vi "vPage_9237x1_CHx4.vi"() -> ()   [LabVIEW 2022 SP3]
uses:
  <vilib>/Utility/sysdir.llb/System Directory Type.ctl
panel:
  in  "Show_FFT":bool
  out "C2":i32
  out "DAQ Stoped":bool
  out "C1":i32
  in  "SW \n(C1)":bool[](array[boolean])=[TRUE, TRUE, TRUE, TRUE, TRUE, TRUE, TRUE, TRUE]
  in  "Sample \nto Read":i32=2000
  in  "Sample\nRate":dbl=2000.0
  in  "¸ê®Æ§¨\nµù°O>":string
  in  "Enable Saving":bool
  in  "Stop":bool
  out "C1-Save":bool
  out "C1-Trigger":bool
  out "C1-All":dynamicdata(graph)
  out "C1-0":dynamicdata(graph)
  out "C1-2":dynamicdata(graph)
  out "C1-1":dynamicdata(graph)
  out "C1-3":dynamicdata(graph)
  # "使用前請先確認 \nDAQ 擷取卡設定"
  # "本頁畫面顯示為 觸發後訊號"
  # "FFT Filter by useing High-pass with Lower Cut-Off (Hz)"
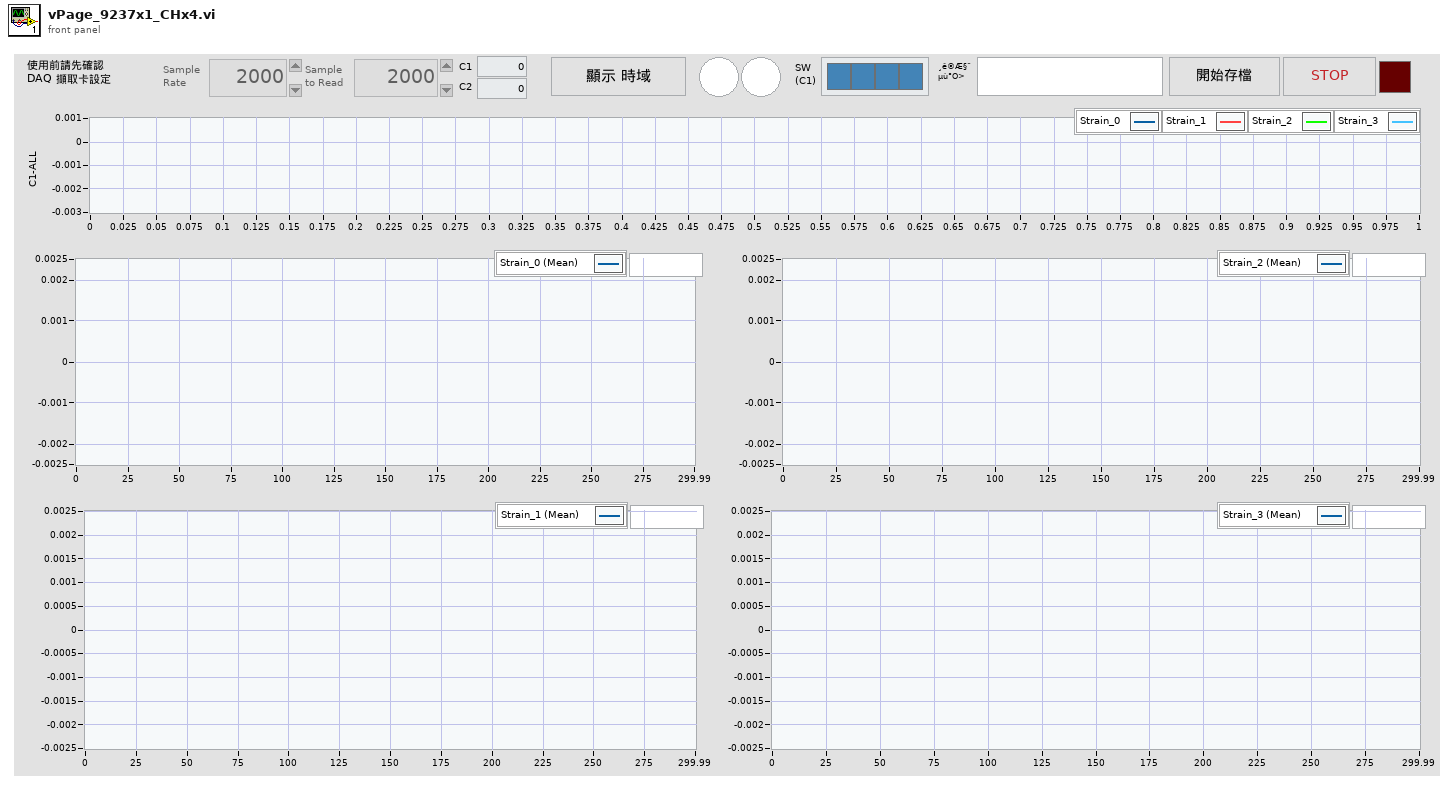
[diagram p1: front panel]
types:
  T1 = enum8{"Enabled", "Disabled", "Disabled and Grayed Out"}
  T2 = typedef "System Directory Type.ctl" = i32
  T3 = cluster{"task out":refnum<k21>, "data":dynamicdata}
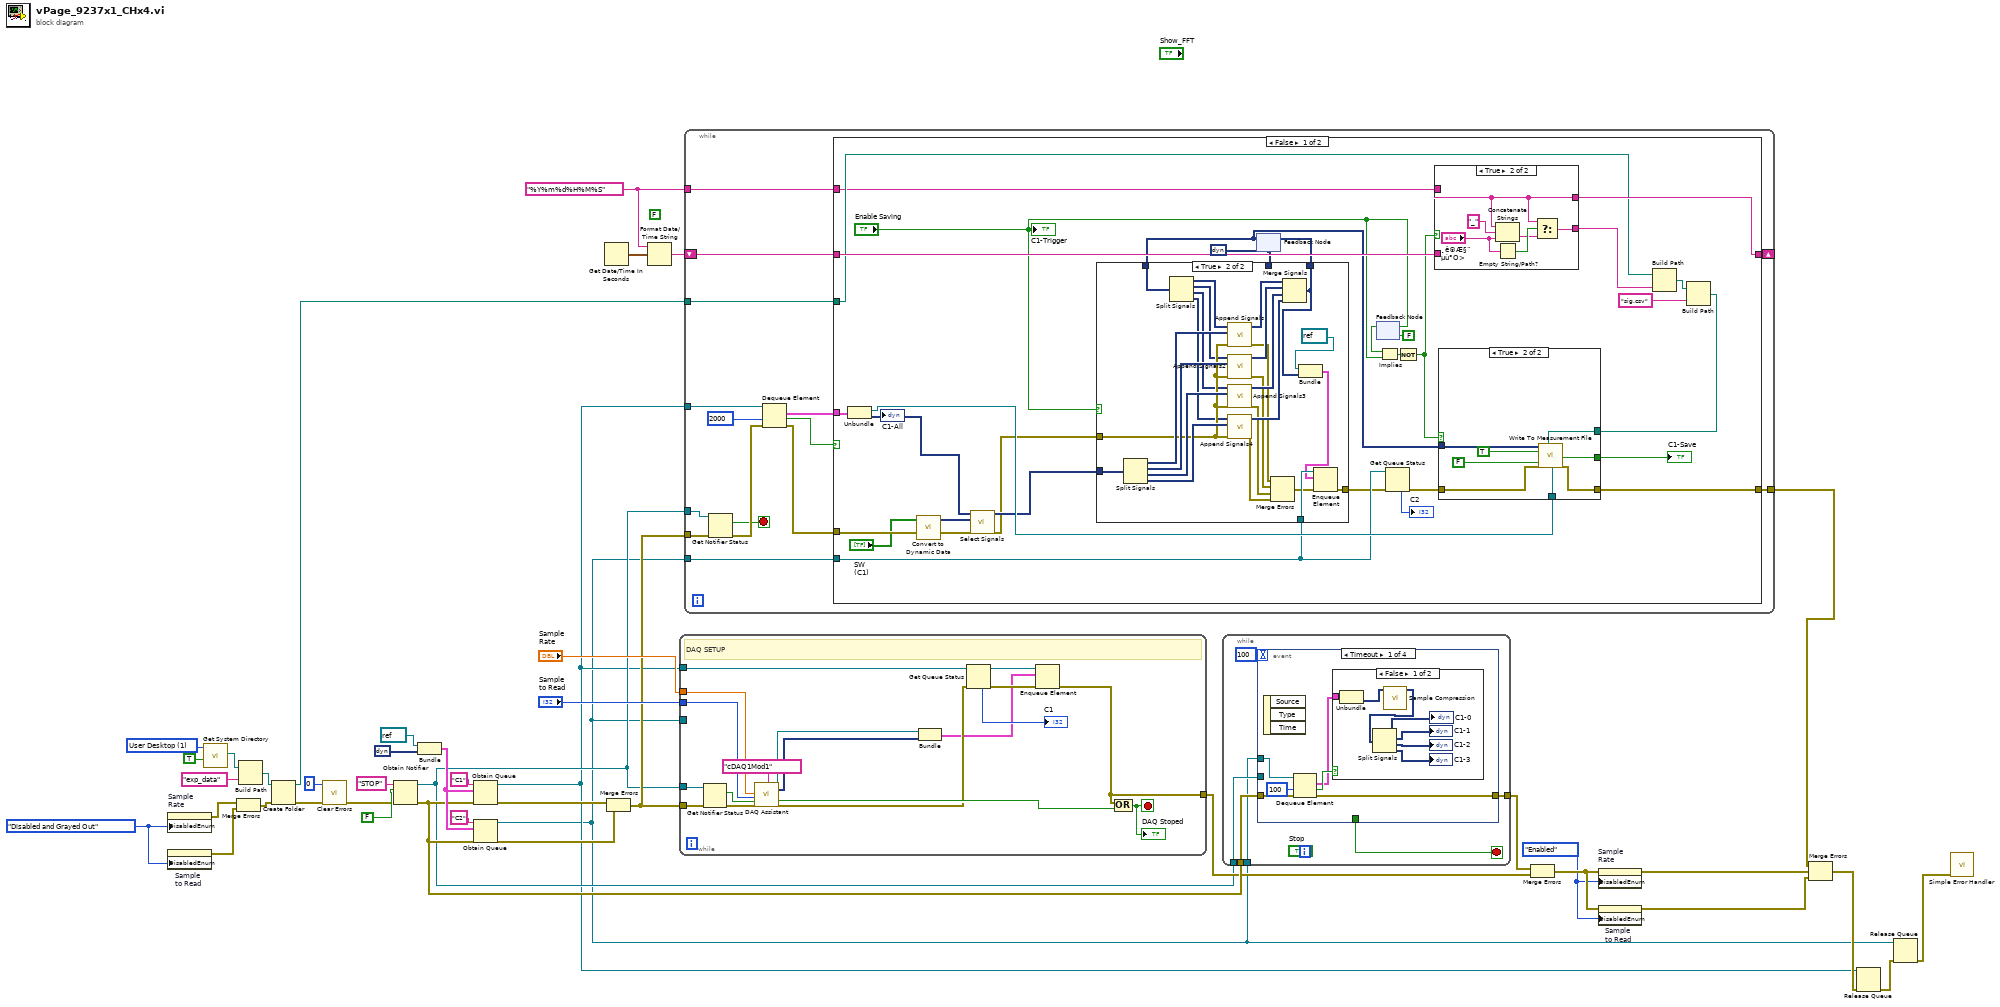
[diagram p0: block diagram]
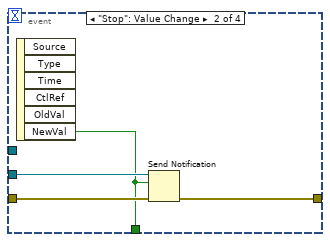
[diagram p3: hidden frame]
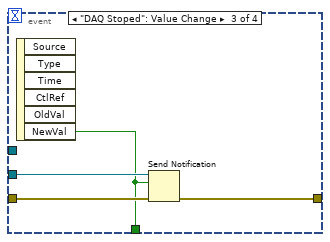
[diagram p4: hidden frame]
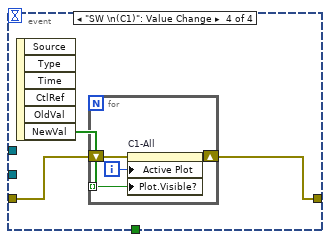
[diagram p5: hidden frame]
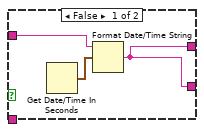
[diagram p8: hidden frame]
diagram:
  (unwired) FALSE
  w9 = T1."Enabled" ("Disabled")
  w14 = T1."Disabled and Grayed Out" ("Disabled")
  w15 = "%Y%m%d%H%M%S" ("time format string (%c)")
  w25 = T2 1 items=["User Home"=0, "User Desktop"=1, "User Documents"=2, "User Application Data"=3, "User Preferences"=4, "User Temporary"=5, "Public Documents"=6, "Public Application Data"=7, "Public Preferences"=8, "Public Cache"=13, "System Core Libraries"=9, "System Installed Libraries"=10, "Application Files"=11, "Boot Volume Root"=12] ("system directory type")
  n1 = property on="Sample\nRate" class="DigNum (strict)"("DisabledEnum"=w14) -> (error out=w13:errorcluster)  [unwired: 2 in, 1 out]
  n2 = property on="Sample \nto Read" class="DigNum (strict)"("DisabledEnum"=w14) -> (error out=w11:errorcluster)  [unwired: 2 in, 1 out]
  n3 = call <vilib>:"Get System Directory.vi"("create directory if not found? (F)"=TRUE, "system directory type"=w25) -> ("system directory"=w27:path)  [unwired: 9 in]
  n4 = Merge Errors(w13, w11) -> (w12:errorcluster)
  n5 = Build Path(base path=w27, name or relative path="exp_data") -> (appended path=w21:path)
  n6 = Create Folder(path (use dialog)=w21, error in=w12) -> (created path=w20:path, error out=w23:errorcluster)  [unwired: 1 in, 1 out]
  n7 = call <vilib>:"Clear Errors.vi"("error in (no error)"=w23, "specific error code to clear (0: all)"=0) -> ("error out"=w22:errorcluster)  [unwired: 4 in, 1 out]
  n8 = Obtain Notifier(name (unnamed)="STOP", notification data type=FALSE, error in (no error)=w22) -> (notifier out=w16:refnum<notifier>, error out=w19:errorcluster)  [unwired: 1 in, 1 out]
  n9 = Bundle("task out"=refnum<k21> refnum, "data"=dynamicdata []) -> (w32:T3)  [unwired: 1 in]
  n10 = Obtain Queue(name (unnamed)="C1", element data type=w32, error in (no error)=w19) -> (queue out=w2:refnum<queue>, error out=w42:errorcluster)  [unwired: 2 in, 1 out]
  n11 = Obtain Queue(name (unnamed)="C2", element data type=w32, error in (no error)=w19) -> (queue out=w1:refnum<queue>, error out=w41:errorcluster)  [unwired: 2 in, 1 out]
  n12 = Get Date/Time In Seconds() -> (seconds since 1Jan1904=w30:timestamp)
  n13 = Merge Errors(w42, w41) -> (w31:errorcluster)
  n14 = Format Date/Time String(time format string (%c)=w15, seconds (now)=w30) -> (date/time string=w29:string)  [unwired: 1 in]
  n15 = while {
    tunnel: [w55] -> w17
    tunnel: w1 -> [_]
    tunnel: w2 -> [w52]
    tunnel: w31 -> [w51]
    tunnel: w16 -> [w50]
    tunnel: "Sample \nto Read" -> [w46]
    tunnel: "Sample\nRate" -> [w45]
    stop <- w53 stop-if-true
    # "DAQ SETUP"
    n16 = Get Notifier Status(notifier=w50, error in (no error)=w51) -> (current notification=w59:bool, error out=w60:errorcluster)  [unwired: 3 out]
    n17 = call "DAQ Assistant"("rate"=w45, "number of samples"=w46, "error in"=w60, "stop (F)"=w59, "device name"=tag "cDAQ1Mod1") -> ("task out"=w48:refnum<k21>, "data"=w44:dynamicdata, "stopped"=w58:bool, "error out"=w56:errorcluster)  [unwired: 11 in]
    n18 = Bundle("task out"=w48, "data"=w44) -> (w47:T3)  [unwired: 1 in]
    n19 = Get Queue Status(queue=w52, error in (no error)=w56) -> (queue out=w49:refnum<queue>, error out=w57:errorcluster, # elements in queue=→"C1":i32)  [unwired: 1 in, 5 out]
    n20 = Enqueue Element(queue=w49, element=w47, error in (no error)=w57) -> (error out=w55:errorcluster)  [unwired: 1 in, 2 out]
    n21 = Compound Arithmetic op=OR(w55, w58) -> (w53:bool)
    "DAQ Stoped" <- w53
  }
  n22 = while {
    tunnel: w31 -> [w75]
    tunnel: w16 -> [w73]
    tunnel: w2 -> [w72]
    tunnel: w1 -> [w61]
    shift-right: [w66] -> _
    shift-left: w29 -> [w67]
    tunnel: w20 -> [w65]
    tunnel: [w64] -> w3
    tunnel: w15 -> [w62]
    stop <- w63 stop-if-true
    n23 = Get Notifier Status(notifier=w73, error in (no error)=w75) -> (current notification=w63:bool, error out=w74:errorcluster)  [unwired: 3 out]
    n24 = Dequeue Element(queue=w72, timeout in ms (-1)=2000, error in (no error)=w74) -> (element=w69:T3, timed out?=w70:bool, error out=w68:errorcluster)  [unwired: 1 out]
    n25 = case shown="False" w70 {
      tunnel: w69 -> [w105 _]
      tunnel: w68 -> [w104 w151]
      tunnel: w67 -> [w100 w152]
      tunnel: [w99 w152] -> w66
      tunnel: w65 -> [w98 _]
      tunnel: [w80 w151] -> w64
      tunnel: w62 -> [w90 _]
      tunnel: w61 -> [w79 _]
      frame False {
        w89 = dynamicdata [] ("Waveform Graph")
        n26 = Unbundle(w105) -> ("task out"=w102:refnum<k21>, "data"=w103:dynamicdata)
        "C1-All" <- w103
        n27 = call "Convert to Dynamic Data"("Array"="SW \n(C1)") -> ("Dynamic Data Type"=w92:dynamicdata)  [unwired: 3 in]
        n28 = call "Select Signals"("error in (no error)"=w104, "Selector Input"=w92, "Signals"=w103) -> ("error out"=w87:errorcluster, "Signal Out"=w101:dynamicdata)  [unwired: 7 in]
        n29 = feedback #1(w89) -> (w81:dynamicdata)
        n30 = case shown="True" "Enable Saving" {
          tunnel: w101 -> [_ w141]
          tunnel: w87 -> [w115 w136]
          tunnel: w81 -> [_ w123]
          tunnel: [w116 w121] -> w82
          tunnel: w89 -> [w116 _]
          tunnel: [w115 w117] -> w78
          tunnel: w79 -> [_ w120]
          frame False {
          }
          frame True {
            n31 = Split Signals(w141) -> (w137:dynamicdata, w138:dynamicdata, w139:dynamicdata, w140:dynamicdata)  [unwired: 4 in]
            n32 = Split Signals(w123) -> (w128:dynamicdata, w129:dynamicdata, w130:dynamicdata, w131:dynamicdata)  [unwired: 4 in]
            n33 = call "Append Signals"("error in (no error)"=w136, "Input Signal B"=w137, "Input Signal A"=w128) -> ("error out"=w127:errorcluster, "Appended Signals"=w135:dynamicdata)  [unwired: 7 in]
            n34 = call "Append Signals2"("error in (no error)"=w136, "Input Signal B"=w138, "Input Signal A"=w129) -> ("error out"=w126:errorcluster, "Appended Signals"=w134:dynamicdata)  [unwired: 7 in]
            n35 = call "Append Signals3"("error in (no error)"=w136, "Input Signal B"=w139, "Input Signal A"=w130) -> ("error out"=w125:errorcluster, "Appended Signals"=w133:dynamicdata)  [unwired: 7 in]
            n36 = call "Append Signals4"("error in (no error)"=w136, "Input Signal B"=w140, "Input Signal A"=w131) -> ("error out"=w124:errorcluster, "Appended Signals"=w132:dynamicdata)  [unwired: 7 in]
            n37 = Merge Errors(w127, w126, w125, w124) -> (w119:errorcluster)
            n38 = Merge Signals(w135, w134, w133, w132) -> (w121:dynamicdata)
            n39 = Bundle("task out"=refnum<k21> refnum, w121) -> (w118:cluster{"task out":refnum<k21>, dynamicdata})  [unwired: 1 in]
            n40 = Enqueue Element(queue=w120, element=w118, error in (no error)=w119) -> (error out=w117:errorcluster)  [unwired: 1 in, 2 out]
          }
        }
        n41 = feedback-in #1(w82) -> ()
        n42 = feedback-in #2("Enable Saving") -> ()
        n43 = feedback #2(FALSE ("Enable Saving")) -> (w86:bool)
        n44 = Implies(1:"Enable Saving", 2:w86) -> (0:w88:bool)
        n45 = Get Queue Status(queue=w79, error in (no error)=w78) -> (error out=w77:errorcluster, # elements in queue=→"C2":i32)  [unwired: 1 in, 6 out]
        n46 = Not(x=w88) -> (.not. x?=w83:bool)
        n47 = case shown="True" w83 {
          tunnel: [w142 w145] -> w99
          tunnel: w100 -> [_ w145]
          tunnel: [w142 w147] -> w91
          tunnel: w90 -> [w143 _]
          frame False {
            n48 = Get Date/Time In Seconds() -> (seconds since 1Jan1904=w144:timestamp)
            n49 = Format Date/Time String(time format string (%c)=w143, seconds (now)=w144) -> (date/time string=w142:string)  [unwired: 1 in]
          }
          frame True {
            n50 = Concatenate Strings(w145, "_" ("string"), "¸ê®Æ§¨\nµù°O>") -> (w148:string)
            n51 = Empty String/Path?(string/path="¸ê®Æ§¨\nµù°O>") -> (empty?=w149:bool)
            n52 = Select(t=w145, s=w149, f=w148) -> (s? t:f=w147:string)
          }
        }
        n53 = Build Path(base path=w98, name or relative path=w91) -> (appended path=w97:path)
        n54 = Build Path(base path=w97, name or relative path="sig.csv") -> (appended path=w95:path)
        n55 = case shown="True" w83 {
          tunnel: w102 -> [_ w114]
          tunnel: w95 -> [_ w113]
          tunnel: [_ w112] -> w94
          tunnel: w81 -> [_ w110]
          tunnel: w77 -> [w106 w108]
          tunnel: [w106 w107] -> w80
          frame False {
          }
          frame True {
            n56 = call "Write To Measurement File"("Signals"=w110, "Enable"=TRUE, "new_file"=FALSE, "error in (no error)"=w108, "Filename"=w113, "DAQmx Task"=w114) -> ("Saving Data"=w112:bool, "error out"=w107:errorcluster)  [unwired: 11 in, 1 out]
          }
        }
        "C1-Save" <- w94
        "C1-Trigger" <- "Enable Saving"
      }
      frame True {
      }
    }
  }
  n57 = while {
    tunnel: w19 -> [w158]
    tunnel: [w157] -> w18
    tunnel: w16 -> [w156]
    tunnel: w1 -> [w153]
    stop <- w155 stop-if-true
    n58 = event shown="[0] Timeout" {
      selector: _ -> [_ _ _ _]
      dyn-events: _ -> [_ _ _ _]
      timeout: 100 -> [_ _ _ _]
      tunnel: w158 -> [w163 w175 w179 w182]
      tunnel: [w162 w174 w178 w181] -> w157
      tunnel: w156 -> [_ w173 w177 _]
      tunnel: [_ w172 w176 _] -> w155
      tunnel: w153 -> [w164 _ _ _]
      event Timeout {
        n59 = event-data() -> ()  [unwired: 1 in, 3 out]
        n60 = Dequeue Element(queue=w164, timeout in ms (-1)=100, error in (no error)=w163) -> (element=w159:T3, timed out?=w160:bool, error out=w162:errorcluster)  [unwired: 1 out]
        n61 = case shown="False" w160 {
          tunnel: w159 -> [w171 _]
          frame False {
            n62 = Unbundle(w171) -> ("data"=w166:dynamicdata)  [unwired: 1 out]
            n63 = call "Sample Compression"("Signals"=w166) -> ("Mean"=w165:dynamicdata)  [unwired: 8 in, 2 out]
            n64 = Split Signals(w165) -> (→"C1-0":dynamicdata, →"C1-1":dynamicdata, →"C1-2":dynamicdata, →"C1-3":dynamicdata)  [unwired: 4 in]
          }
          frame True {
          }
        }
      }
      event "Stop": Value Change {
        n65 = event-data() -> ("NewVal"=w172:bool)  [unwired: 1 in, 5 out]
        n66 = Send Notification(notification=w172, notifier=w173, error in (no error)=w175) -> (error out=w174:errorcluster)  [unwired: 1 out]
      }
      event "DAQ Stoped": Value Change {
        n67 = event-data() -> ("NewVal"=w176:bool)  [unwired: 1 in, 5 out]
        n68 = Send Notification(notification=w176, notifier=w177, error in (no error)=w179) -> (error out=w178:errorcluster)  [unwired: 1 out]
      }
      event "SW \n(C1)": Value Change {
        n69 = event-data() -> ("NewVal"=w180:bool[])  [unwired: 1 in, 5 out]
        n70 = for {
          shift-right: [w185] -> w181
          shift-left: w182 -> [w186]
          tunnel: w180 -> [w183] mode=indexing
          i -> [w184]
          n71 = property on="C1-All" class="WFGraph (strict)"(error in=w186, "Active Plot"=w184, "Plot.Visible?"=w183) -> (error out=w185:errorcluster)  [unwired: 1 in, 1 out]
        }
      }
    }
  }
  n72 = Merge Errors(w18, w17) -> (w10:errorcluster)
  n73 = property on="Sample\nRate" class="DigNum (strict)"(error in=w10, "DisabledEnum"=w9) -> (error out=w8:errorcluster)  [unwired: 1 in, 1 out]
  n74 = property on="Sample \nto Read" class="DigNum (strict)"(error in=w10, "DisabledEnum"=w9) -> (error out=w7:errorcluster)  [unwired: 1 in, 1 out]
  n75 = Merge Errors(w3, w8, w7) -> (w4:errorcluster)
  n76 = Release Queue(queue=w2, error in (no error)=w4) -> (error out=w5:errorcluster)  [unwired: 1 in, 2 out]
  n77 = Release Queue(queue=w1, error in (no error)=w5) -> (error out=w6:errorcluster)  [unwired: 1 in, 2 out]
  n78 = call <vilib>:"Simple Error Handler.vi"("error in (no error)"=w6) -> ()  [unwired: 4 in, 5 out]
